vi "Find Endpoint Configuration Section.vi"(8 "error in":errorcluster, 11 "slsc switch custom device in":T1 format="%.0x") -> (0 "error out":errorcluster, 2 "endpoint configuration":T1 format="%.0x", 3 "slsc switch custom device out":T1 format="%.0x")   [LabVIEW 2020, in "SLSC Switch Scripting.lvlib"]
doc: "Returns the Endpoint Configuration section for the custom device."
uses:
  SLSC Switch Scripting.lvlib
  <vilib>/NI VeriStand/Custom Device API/Custom Device Item Ref.ctl
  NationalInstruments.VeriStand.SystemDefinitionAPI
  SLSC Scripting Constants.vi
  <vilib>/NI VeriStand/Custom Device API/Custom Device API.lvlib
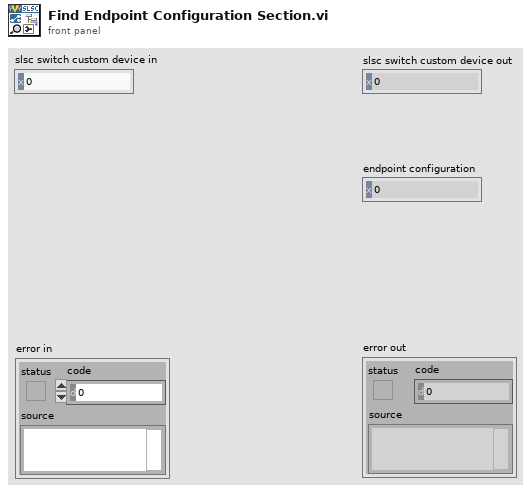
[diagram p1: front panel]
types:
  T1 = typedef "Custom Device API.lvlib/Custom Device Item Ref.ctl" = u64
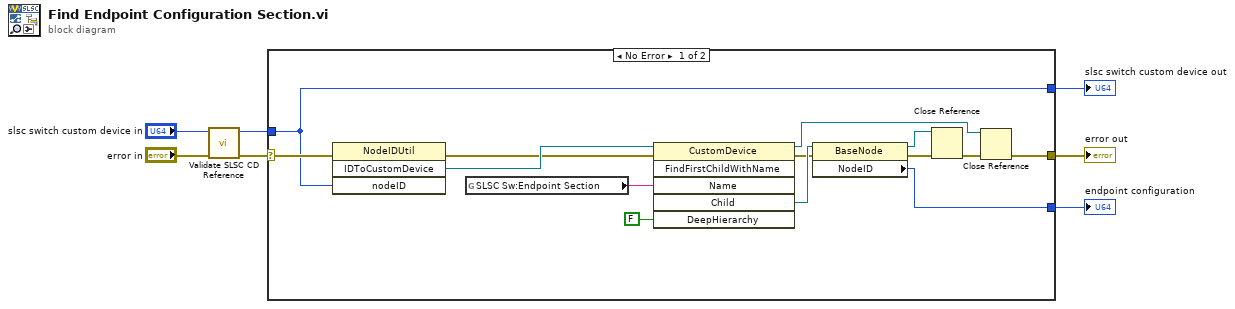
[diagram p0: block diagram]
diagram:
  n1 = call "Validate SLSC CD Reference.vi"("error in"="error in", "slsc switch custom device in"="slsc switch custom device in") -> ("error out"=w3:errorcluster, "slsc switch custom device out"=w1:T1)  [unwired: 8 in]
  n2 = case shown="No Error" w3 {
    selector: w3 -> [w15 w23]
    tunnel: w1 -> [w8 w22]
    tunnel: [w8 w22] -> w7
    tunnel: [w9 w23] -> w6
    tunnel: [w17 _] -> w4
    frame No Error {
      n3 = invoke class="NodeIDUtil" method="IDToCustomDevice"(error in=w15, "nodeID"=w8) -> (error out=w14:errorcluster, "IDToCustomDevice"=w16:refnum<k24>)  [unwired: 2 in, 2 out]
      n4 = global read "SLSC Scripting Constants.vi" "SLSC Sw:Endpoint Section"() -> (w21:string)
      n5 = invoke class="CustomDevice" method="FindFirstChildWithName"(reference=w16, error in=w14, "Name"=w21, "DeepHierarchy"=FALSE) -> (reference out=w10:refnum<k24>, error out=w19:errorcluster, "Child"=w20:refnum<k24>)  [unwired: 2 in, 3 out]
      n6 = property class="BaseNode"(reference=w20, error in=w19) -> (reference out=w12:refnum<k24>, error out=w13:errorcluster, "NodeID"=w17:u64)
      n7 = Close Reference(reference=w12, error in (no error)=w13) -> (error out=w11:errorcluster)
      n8 = Close Reference(reference=w10, error in (no error)=w11) -> (error out=w9:errorcluster)
    }
    frame Error {
    }
  }
  "slsc switch custom device out" <- w7
  "endpoint configuration" <- w4
  "error out" <- w6
